vi "Read.vi"(8 "error in (no error)":errorcluster, 10 "ReadElements":u32=10000, 11 "AODAcq in":refnum<class "AODAcq.lvclass">) -> (0 "error out":errorcluster, 1 "TemporalData":waveform(dbl)[](array[waveform]), 2 "ImData":waveform(i32)[](array[waveform]), 3 "AODAcq out":refnum<class "AODAcq.lvclass">, 4 "ReadFraction":dbl, 5 "MotionData":waveform(i32)[](array[waveform]), 6 "Done":bool)   [LabVIEW 2011, in "AODAcq.lvclass"]
uses:
  AODAcq.lvclass
  FPGA_Control/FPGAState.ctl
  AODAcq.lvclass/AODAcq.ctl
  <vilib>/rvi/interface/RandomDataEmulation/nirviRandomDataDMAMethods.vi
  <vilib>/rvi/interface/RandomDataEmulation/niFpgaReadControlTemplate.vi
  <vilib>/rvi/interface/nirviMethod/nirviMethod.xnode
  FPGA_Control/AODRef.ctl
  FPGA_Control/AOD Control (FPGA).vi
  <vilib>/rvi/interface/nirviReadWriteControl/nirviReadWriteControl.xnode
panel:
  out "PMT Transfers":i32
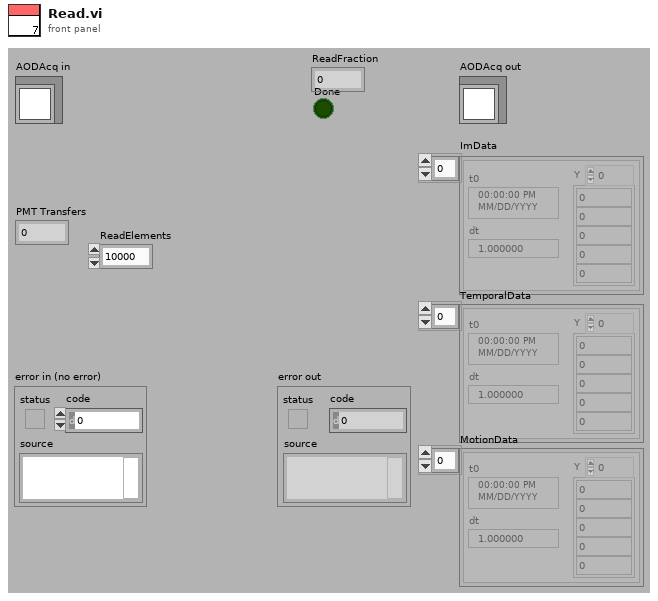
[diagram p1: front panel]
types:
  T1 = typedef "FPGAState.ctl" = enum16{"Idle", "Arm Scan", "Scan", "End Scan"}
  T2 = typedef "AODRef.ctl" = refnum<k20>
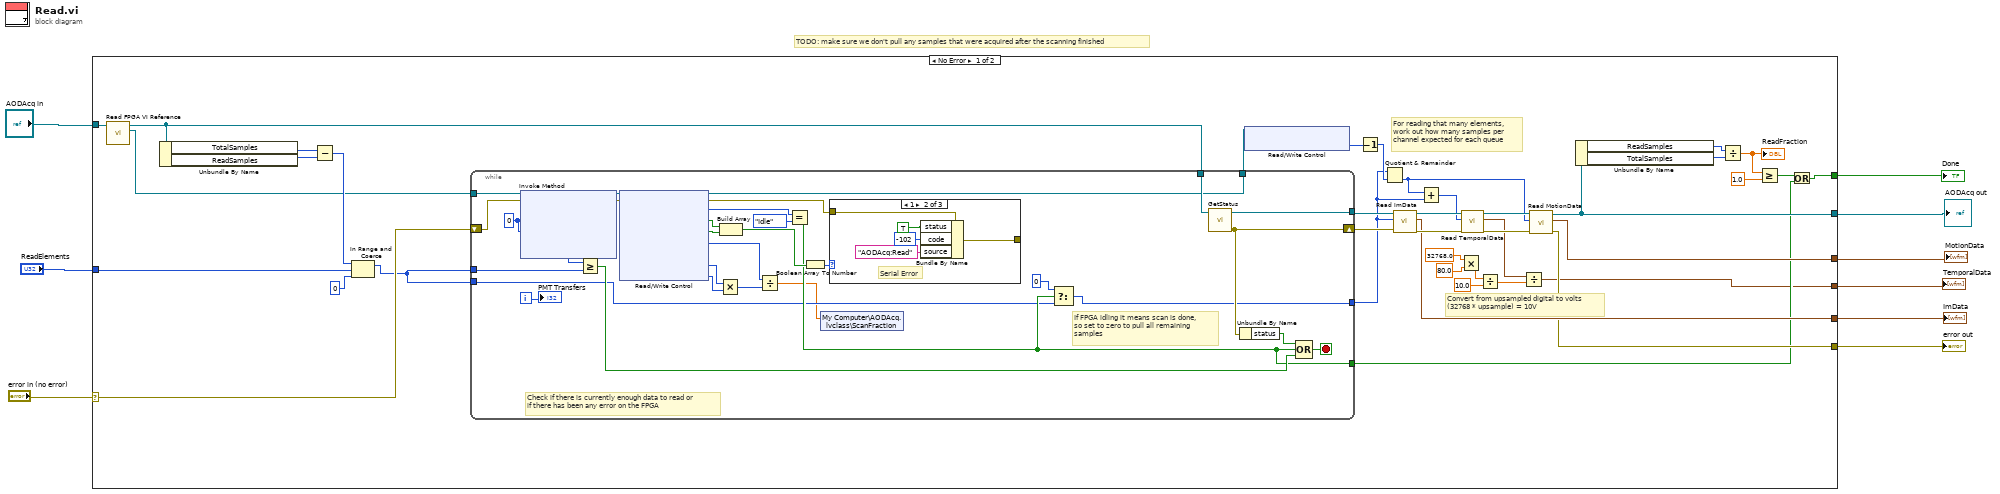
[diagram p0: block diagram]
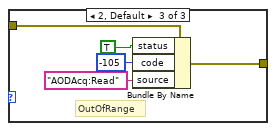
[diagram p3: hidden frame]
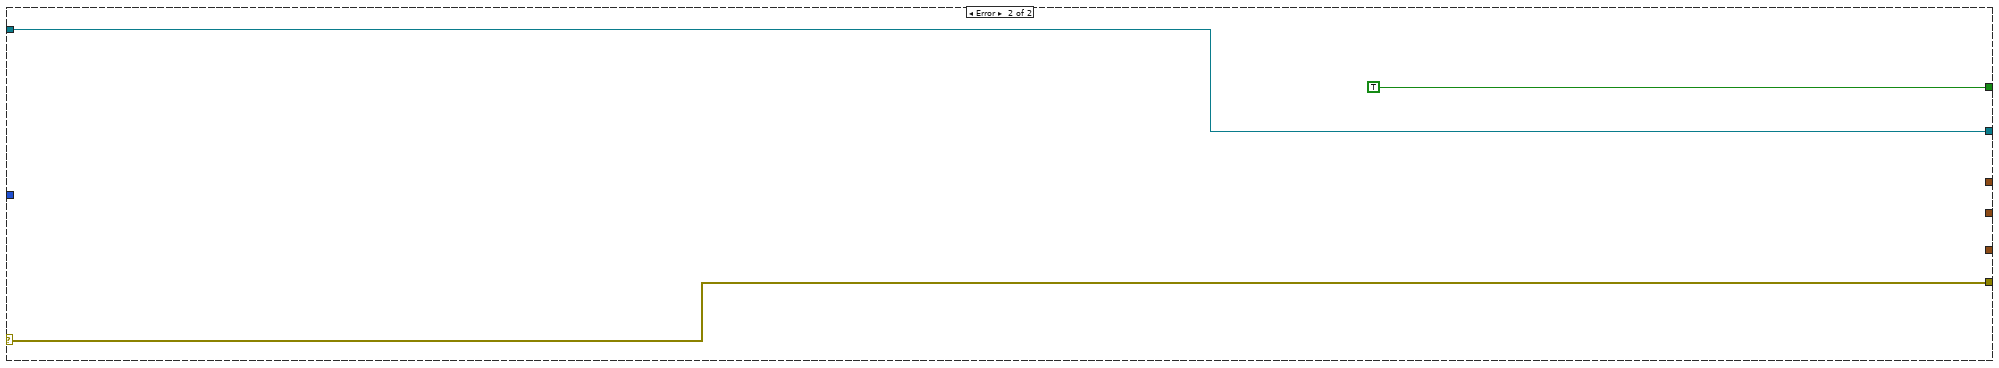
[diagram p4: hidden frame]
diagram:
  # "TODO: make sure we don't pull any samples that were acquired after the scanning finished"
  n1 = case shown="No Error" "error in (no error)" {
    selector: "error in (no error)" -> [w44 w94]
    tunnel: [w29 w94] -> w8
    tunnel: [w35 w93] -> w6
    tunnel: "AODAcq in" -> [w49 w93]
    tunnel: "ReadElements" -> [w46 _]
    tunnel: [w30 _] -> w4
    tunnel: [w17 _] -> w3
    tunnel: [w28 _] -> w2
    tunnel: [w25 TRUE] -> w1
    frame No Error {
      # "Convert from upsampled digital to volts\n(32768 * upsample) = 10V"
      # "For reading that many elements,\nwork out how many samples per\nchannel expected for each queue"
      n2 = call-dynamic "Read FPGA VI Reference.vi"("AODAcq in"=w49) -> ("FPGA VI Reference"=w11:T2, "AODAcq out"=w43:refnum<class "AODAcq.lvclass">)  [unwired: 8 in, 1 out]
      n3 = Unbundle By Name(w43) -> ("TotalSamples"=w45:u64, "ReadSamples"=w36:u64)
      n4 = Subtract(x=w45, y=w36) -> (x-y=w47:u64)
      n5 = In Range and Coerce(upper limit=w47, x=w46, lower limit=u32 0) -> (coerced(x)=w10:u64)  [unwired: 1 out]
      n6 = while {
        tunnel: w10 -> [w66]
        tunnel: w11 -> [w79]
        tunnel: [w56] -> w21
        tunnel: [w50] -> w24
        tunnel: w43 -> [w63]
        shift-right: [w61] -> w40
        shift-left: w44 -> [w76]
        tunnel: [w60] -> w37
        tunnel: [w59] -> w26
        tunnel: w10 -> [w57]
        i -> [w77]
        stop <- w78 stop-if-true
        w80 = u32 0 ("Number of Elements")
        # "If FPGA idling it means scan is done, \nso set to zero to pull all remaining\nsamples"
        # "Check if there is currently enough data to read or \nif there has been any error on the FPGA"
        n7 = xnode "Invoke Method"("FPGA VI Reference In"=w79, "error in"=w76, "Number of Elements"=w80, "Timeout (ms)"=w80) -> ("FPGA VI Reference Out"=w70:T2, "error out"=w71:errorcluster, "Elements Remaining"=w67:u32)  [unwired: 1 out]
        n8 = Greater Or Equal?(x=w67, y=w66) -> (x >= y?=w64:bool)
        n9 = xnode "Read/Write Control"("FPGA VI Reference In"=w70, "error in"=w71) -> ("FPGA VI Reference Out"=w50:T2, "error out"=w65:errorcluster, "Status.State"=w68:T1, "Status.Serial error"=w75:bool, "Status.OutOfRange"=w74:bool, "Status.PointNum"=w51:u32, "Scan.NumPoints"=w55:u32, "Scan.NumReps"=w54:i32)  [unwired: 1 out]
        n10 = Multiply(x=w55, y=w54) -> (x*y=w53:u32)
        n11 = Build Array(w75, w74) -> (w73:bool[])
        n12 = Divide(x=w51, y=w53) -> (x/y=w52:dbl)
        n13 = Equal?(x=w68, y=FPGAState."Idle" ("x")) -> (x = y?=w59:bool)
        n14 = Boolean Array To Number(Boolean array=w73) -> (number=w72:u32)
        n15 = shared-variable "My Computer\\AODAcq.lvclass\\ScanFraction"(w52) -> ()  [unwired: 1 in, 1 out]
        n16 = case shown="1" w72 {
          tunnel: [w81 w83 w88] -> _
          tunnel: w65 -> [w81 w82 w87]
          frame 0 {
          }
          frame 1 {
            # "Serial Error"
            n17 = Bundle By Name(cluster=w82, "status"=TRUE, "code"=-102, "source"="AODAcq:Read") -> (w83:errorcluster)
          }
          frame 2, Default {
            # "OutOfRange"
            n18 = Bundle By Name(cluster=w87, "status"=TRUE, "code"=-105, "source"="AODAcq:Read") -> (w88:errorcluster)
          }
        }
        n19 = Select(t=u64 0, s=w59, f=w57) -> (s? t:f=w56:u64)
        n20 = call-dynamic "GetStatus.vi"("AODAcq in"=w63) -> ("error out"=w61:errorcluster, "AODAcq out"=w60:refnum<class "AODAcq.lvclass">)  [unwired: 8 in, 1 out]
        n21 = Unbundle By Name(w61) -> ("status"=w62:bool)
        n22 = Compound Arithmetic op=OR(w62, w59, w64) -> (w78:bool)
        "PMT Transfers" <- w77
      }
      n23 = xnode "Read/Write Control"("FPGA VI Reference In"=w24) -> ("Scan.Motion Increment"=w23:u32)  [unwired: 1 in, 2 out]
      n24 = Decrement(x=w23) -> (x-1=w22:u32)
      n25 = Quotient & Remainder(x=w21, y=w22) -> (floor(x/y)=w20:u64)  [unwired: 1 out]
      n26 = call-dynamic "Read ImData.vi"("error in (no error)"=w40, "ReadSize"=w21, "AODAcq in"=w37) -> ("error out"=w39:errorcluster, "ImData"=w30:waveform(i32)[], "AODAcq out"=w42:refnum<class "AODAcq.lvclass">)  [unwired: 6 in]
      n27 = Add(x=w20, y=w21) -> (x+y=w19:u64)
      n28 = Multiply(x=32768.0, y=80.0) -> (x*y=w14:dbl)
      n29 = call-dynamic "Read TemporalData.vi"("error in (no error)"=w39, "ReadSize"=w19, "AODAcq in"=w42) -> ("error out"=w38:errorcluster, "TemporalData"=w18:waveform(i32)[], "AODAcq out"=w41:refnum<class "AODAcq.lvclass">)  [unwired: 6 in]
      n30 = Divide(x=w14, y=10.0) -> (x/y=w12:dbl)
      n31 = Divide(x=w18, y=w12) -> (x/y=w17:waveform(dbl)[])
      n32 = call-dynamic "Read MotionData.vi"("error in (no error)"=w38, "ReadSize"=w20, "AODAcq in"=w41) -> ("error out"=w29:errorcluster, "MotionData"=w28:waveform(i32)[], "AODAcq out"=w35:refnum<class "AODAcq.lvclass">)  [unwired: 6 in]
      n33 = Unbundle By Name(w35) -> ("ReadSamples"=w34:u64, "TotalSamples"=w33:u64)
      n34 = Divide(x=w34, y=w33) -> (x/y=w32:dbl)
      "ReadFraction" <- w32
      n35 = Greater Or Equal?(x=w32, y=1.0) -> (x >= y?=w27:bool)
      n36 = Or(x=w27, y=w26) -> (x .or. y?=w25:bool)
    }
    frame Error {
    }
  }
  "error out" <- w8
  "AODAcq out" <- w6
  "ImData" <- w4
  "TemporalData" <- w3
  "MotionData" <- w2
  "Done" <- w1
